vi "Exit In Place Element Cluster.vi"(0 "Diagram in":refnum<vi>, 5 "Elements":refnum<vi>[](array[refnum]), 7 "Outputs":refnum<vi>[](array[refnum]), 11 "error in (no error)":errorcluster) -> (4 "Diagram out":refnum<vi>, 6 "Cluster":refnum<vi>, 8 "Outputs":refnum<vi>[](array[refnum]), 15 "error out":errorcluster)   [LabVIEW 2015, in "Scripting.lvlib"]
doc: "Exits the In Place Element Structure that owns <B>Diagram in</B>, supplying the structure's owning diagram at <B>Diagram out</B>.\n\n<B>Elements</B> are the terminals to wire to the Bundle by Name node's element terminals.\n\n<B>Cluster</B> is the cluster output terminal of the Bundle by Name node."
uses:
  Scripting.lvlib
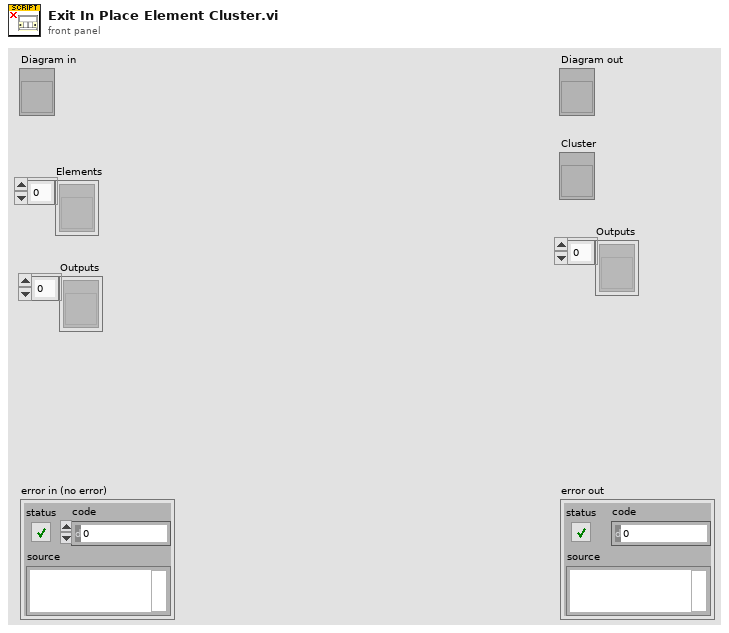
[diagram p1: front panel]
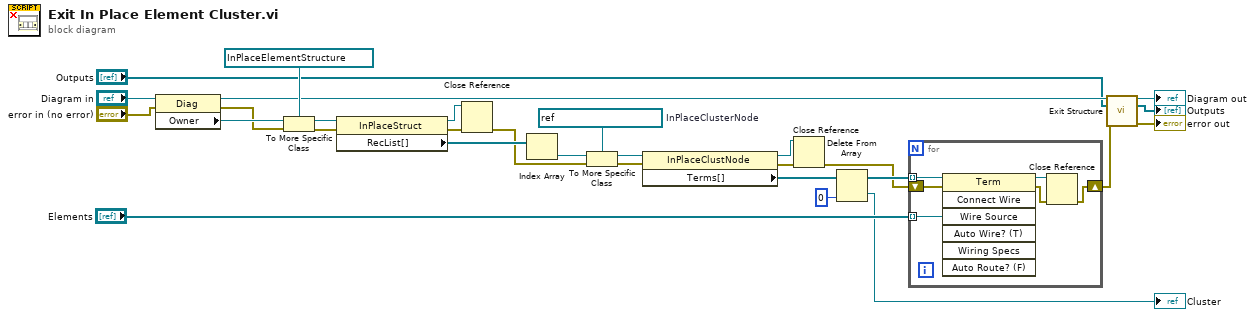
[diagram p0: block diagram]
diagram:
  w10 = refnum<vi> refnum  # InPlaceClusterNode
  n1 = property class="Diag"(reference="Diagram in", error in="error in (no error)") -> (reference out=w18:refnum<vi>, error out=w20:errorcluster, "Owner"=w28:refnum<vi>)
  n2 = To More Specific Class(target class=refnum<vi> refnum ("reference"), reference=w28, error in=w20) -> (specific class reference=w24:refnum<vi>, error out=w26:errorcluster)
  n3 = property class="InPlaceStruct"(reference=w24, error in=w26) -> (reference out=w3:refnum<vi>, error out=w27:errorcluster, "RecList[]"=w25:refnum<vi>[])
  n4 = Close Reference(reference=w3, error in (no error)=w27) -> (error out=w4:errorcluster)
  n5 = Index Array(array=w25) -> (element=w12:refnum<vi>)  [unwired: 1 in]
  n6 = To More Specific Class(target class=w10, reference=w12, error in=w4) -> (specific class reference=w11:refnum<vi>, error out=w13:errorcluster)
  n7 = property class="InPlaceClustNode"(reference=w11, error in=w13) -> (reference out=w1:refnum<vi>, error out=w29:errorcluster, "Terms[]"=w8:refnum<vi>[])
  n8 = Close Reference(reference=w1, error in (no error)=w29) -> (error out=w2:errorcluster)
  n9 = Delete From Array(array=w8, index=0) -> (deleted portion=→"Cluster":refnum<vi>, array with subset deleted=w7:refnum<vi>[])  [unwired: 1 in]
  n10 = for {
    tunnel: "Elements" -> [w34] mode=indexing
    shift-right: [w31] -> w19
    shift-left: w2 -> [w35]
    tunnel: w7 -> [w32] mode=indexing
    n11 = invoke class="Term" method="Connect Wire"(reference=w32, error in=w35, "Wire Source"=w34) -> (reference out=w30:refnum<vi>, error out=w33:errorcluster)  [unwired: 4 in, 5 out]
    n12 = Close Reference(reference=w30, error in (no error)=w33) -> (error out=w31:errorcluster)
  }
  n13 = call "Exit Structure.vi"("Diagram in"=w18, "Outputs"="Outputs", "error in (no error)"=w19) -> ("Diagram out"=→"Diagram out":refnum<vi>, "Outputs"=→"Outputs":refnum<vi>[], "error out"=→"error out":errorcluster)  [unwired: 10 in]
